vi "Add Stop Condition.vi"(8 "error in (no error)":errorcluster, 11 "I2C waveform info":T1) -> (0 "error out":errorcluster, 3 "I2C waveform info out":T1)   [LabVIEW 2009, in "IDW.lvlib"]
doc: "Adds a Stop (P) condition to the I2C waveform. \n\nTiming parameters that affect this waveform segment's length are: <b>tSU;DAT</b>, <b>tSU;STO</b>, and <b>tBUF</b>"
uses:
  IDW.lvlib
  _Typedefs/Waveform info.ctl
  _Typedefs/Timing - ticks.ctl
  _Typedefs/Default transition action.ctl
  _Typedefs/Bit type.ctl
  _Private/Polymorphics/Change Bit Value - Single.vi
  _Private/Polymorphics/Change Bit Value - Multi.vi
  _Typedefs/Channel Ring.ctl
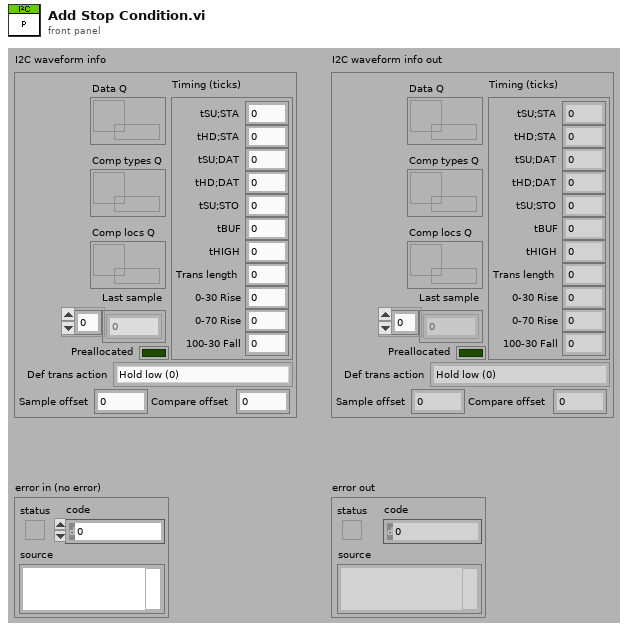
[diagram p1: front panel]
types:
  T1 = typedef "IDW.lvlib/Waveform info.ctl" = cluster{"Last sample":u8[], "Sample offset":u64, "Compare offset":u64, "Timing (ticks)":T2, "Preallocated":bool, "Def trans action":T3, "Data Q":refnum<queue>, "Comp types Q":refnum<queue>, "Comp locs Q":refnum<queue>}
  T2 = typedef "IDW.lvlib/Timing - ticks.ctl" = cluster{"tSU;STA":i32, "tHD;STA":i32, "tSU;DAT":i32, "tHD;DAT":i32, "tSU;STO":i32, "tBUF":i32, "tHIGH":i32, "Trans length":i32, "0-30 Rise":i32, "0-70 Rise":i32, "100-30 Fall":i32}
  T3 = typedef "IDW.lvlib/Default transition action.ctl" = enum16{"Hold low (0)", "Release (Z)", "Set up next value", "Hold previous value", "Preserve tHD;DAT and tSU;DAT"}
  T4 = typedef "IDW.lvlib/Channel ring.ctl" = u16
  T5 = typedef "IDW.lvlib/Channel Ring.ctl" = u16
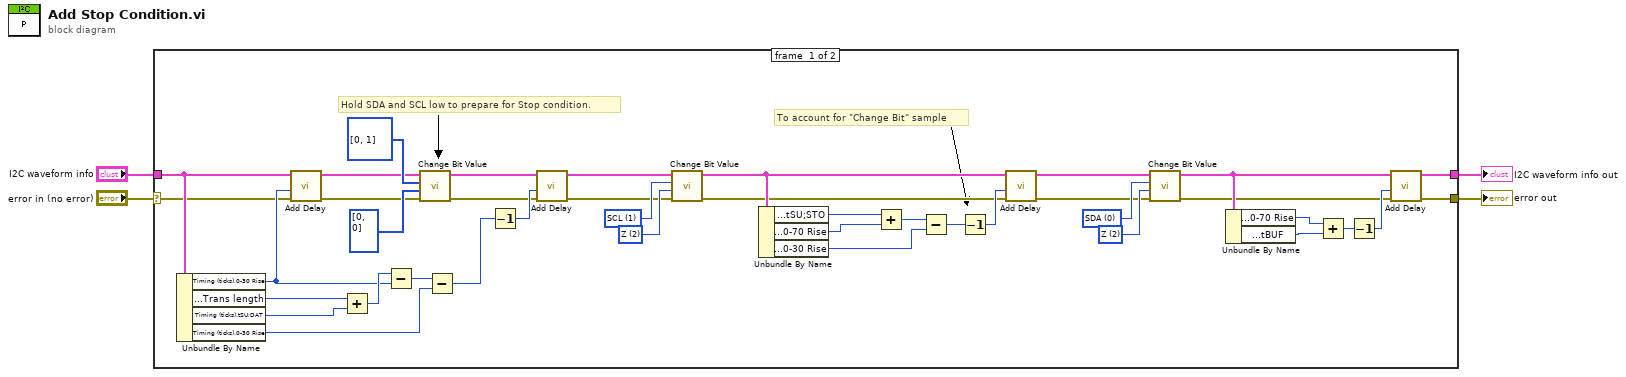
[diagram p0: block diagram]
diagram:
  n1 = case shown="No Error" "error in (no error)" {
    selector: "error in (no error)" -> [w12 w46]
    tunnel: "I2C waveform info" -> [w24 w45]
    tunnel: [w39 w45] -> w3
    tunnel: [w5 w46] -> w1
    frame #0 {
      w34 = T4[] [0, 1] items=["SDA", "SCL"] ("Bits")
      w41 = u8 2 items=["0", "1", "Z", "L", "H", "X", "T", "V"] ("State")
      w42 = T5 0 items=["SDA", "SCL"] ("I2C Ring")
      w44 = u8 2 items=["0", "1", "Z", "L", "H", "X", "T", "V"] ("State")
      w43 = T5 1 items=["SDA", "SCL"] ("I2C Ring")
      w33 = u8[] [0, 0] items=["0", "1", "Z", "L", "H", "X", "T", "V"] ("States")
      # "To account for \"Change Bit\" sample"
      # "Hold SDA and SCL low to prepare for Stop condition."
      n2 = Unbundle By Name(w24) -> ("Timing (ticks).0-30 Rise"=w23:i32, "Timing (ticks).Trans length"=w27:i32, "Timing (ticks).tSU;DAT"=w26:i32, "Timing (ticks).0-30 Rise"=w28:i32)
      n3 = call "Add Delay.vi"("error in (no error)"=w12, "# Samples"=w23, "I2C waveform info"=w24) -> ("error out"=w11:errorcluster, "I2C waveform info out"=w31:T1)  [unwired: 1 in, 6 out]
      n4 = Add(x=w27, y=w26) -> (x+y=w25:i32)
      n5 = Subtract(x=w25, y=w23) -> (x-y=w29:i32)
      n6 = call-poly "Change Bit Value.vi"("error in (no error)"=w11, "States"=w33, "Bits"=w34, "I2C waveform info"=w31) -> ("error out"=w10:errorcluster, "I2C waveform info out"=w30:T1)  [unwired: 6 out]
      n7 = Subtract(x=w29, y=w28) -> (x-y=w22:i32)
      n8 = Decrement(x=w22) -> (x-1=w32:i32)
      n9 = call "Add Delay.vi"("error in (no error)"=w10, "# Samples"=w32, "I2C waveform info"=w30) -> ("error out"=w9:errorcluster, "I2C waveform info out"=w21:T1)  [unwired: 1 in, 6 out]
      n10 = call-poly "Change Bit Value.vi"("error in (no error)"=w9, "State"=w44, "Bit"=w43, "I2C waveform info"=w21) -> ("error out"=w8:errorcluster, "I2C waveform info out"=w38:T1)  [unwired: 6 out]
      n11 = Unbundle By Name(w38) -> ("Timing (ticks).tSU;STO"=w20:i32, "Timing (ticks).0-70 Rise"=w19:i32, "Timing (ticks).0-30 Rise"=w17:i32)
      n12 = Add(x=w20, y=w19) -> (x+y=w18:i32)
      n13 = Subtract(x=w18, y=w17) -> (x-y=w16:i32)
      n14 = Decrement(x=w16) -> (x-1=w36:i32)
      n15 = call "Add Delay.vi"("error in (no error)"=w8, "# Samples"=w36, "I2C waveform info"=w38) -> ("error out"=w7:errorcluster, "I2C waveform info out"=w40:T1)  [unwired: 7 out]
      n16 = call-poly "Change Bit Value.vi"("error in (no error)"=w7, "State"=w41, "Bit"=w42, "I2C waveform info"=w40) -> ("error out"=w6:errorcluster, "I2C waveform info out"=w37:T1)  [unwired: 6 out]
      n17 = Unbundle By Name(w37) -> ("Timing (ticks).0-70 Rise"=w14:i32, "Timing (ticks).tBUF"=w15:i32)
      n18 = Add(x=w14, y=w15) -> (x+y=w13:i32)
      n19 = Decrement(x=w13) -> (x-1=w35:i32)
      n20 = call "Add Delay.vi"("error in (no error)"=w6, "# Samples"=w35, "I2C waveform info"=w37) -> ("error out"=w5:errorcluster, "I2C waveform info out"=w39:T1)  [unwired: 7 out]
    }
    frame #1 {
    }
  }
  "I2C waveform info out" <- w3
  "error out" <- w1
